vi "Take Mean of N Sample.vi"(8 "error in (no error)":errorcluster, 10 "number of samples per channel":i32=20, 11 "Refnum in":refnum<k21>) -> (0 "error out":errorcluster, 1 "Mean Voltage Detected":dbl format="%0.2f", 3 "Refnum out":refnum<k21>)   [LabVIEW 2021]
uses:
  <vilib>/DAQmx/read.llb/DAQmx Read (Analog Wfm 1Chan NSamp).vi
  <vilib>/Analysis/baseanly.llb/Mean (DBL).vi
  <vilib>/DAQmx/miscellaneous.llb/DAQmx Fill In Error Info.vi
  <vilib>/Analysis/NI_AALBase.lvlib
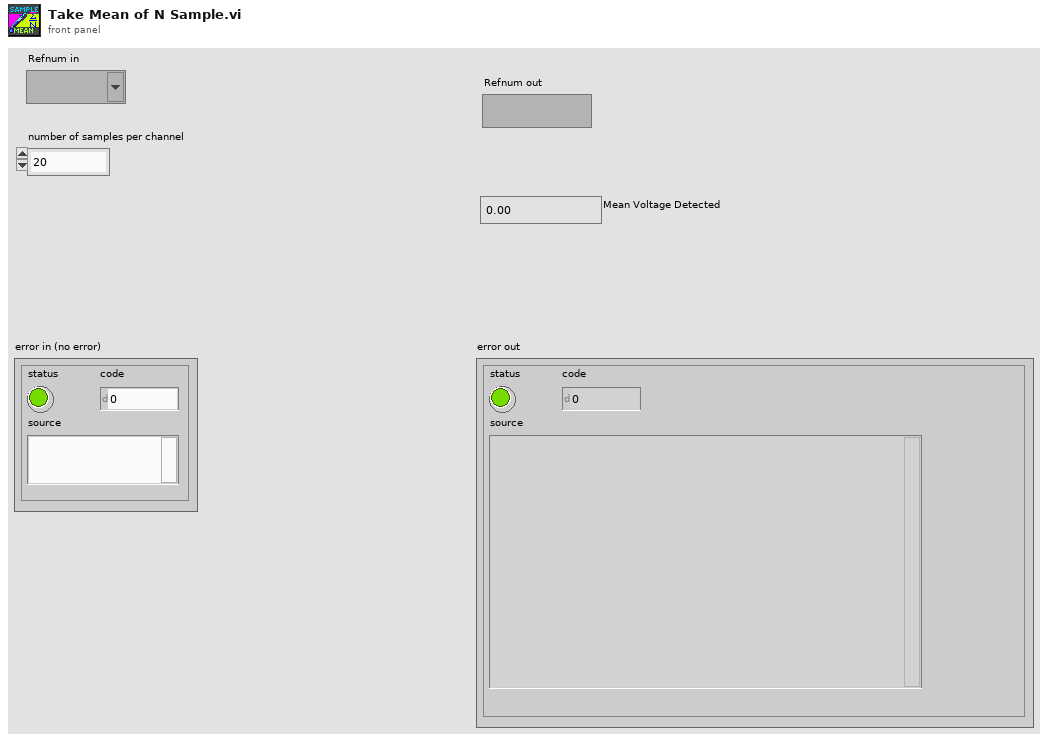
[diagram p1: front panel]
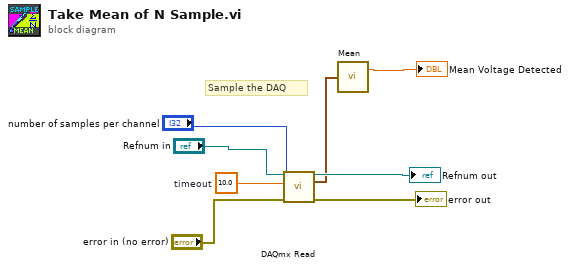
[diagram p0: block diagram]
diagram:
  w4 = 10.0  # timeout
  # "Sample the DAQ"
  n1 = call-poly <vilib>:"DAQmx Read.vi"("task/channels in"="Refnum in", "number of samples per channel"="number of samples per channel", "timeout"=w4, "error in"="error in (no error)") -> ("task out"=→"Refnum out":refnum<k21>, "data"=w5:waveform(dbl), "error out"=→"error out":errorcluster)  [unwired: 9 in]
  n2 = call-poly <vilib>:"Mean.vi"("X"=w5) -> ("mean"=→"Mean Voltage Detected":dbl)  [unwired: 1 out]
